vi "LOAD CELL READ.vi"(8 "error in (no error)":errorcluster, 11 "main ref":T1) -> (0 "error out":errorcluster)   [LabVIEW 2025]
uses:
  v06/controls/LAB-IQ UI Data.ctl
  Traction Loop/Traction Receipe Enum.ctl
  v05/LOAD CELL CODE/New Logic/Load cell Enum.ctl
  <vilib>/Analysis/baseanly.llb/Mean (DBL).vi
  <vilib>/Analysis/5stat.llb/RMS (DBL).vi
  <vilib>/Analysis/Matrix/Numeric/Conversions/Array To Matrix - RA.vi
  <vilib>/Analysis/Matrix/Numeric/Conversions/Matrix To Array - RM.vi
  <vilib>/Analysis/NI_AALBase.lvlib
  <vilib>/ptbypt/NI_PtbyPt.lvlib
  <vilib>/Analysis/NI_AALPro.lvlib
  <vilib>/Analysis/Matrix/NI_Matrix.lvlib
panel:
  out "Fload 3":dbl
  out "Fload 2":dbl
  out "Fload":dbl
  out "Friction":dbl
  out "Load Temp":dbl
  out "Zload":dbl
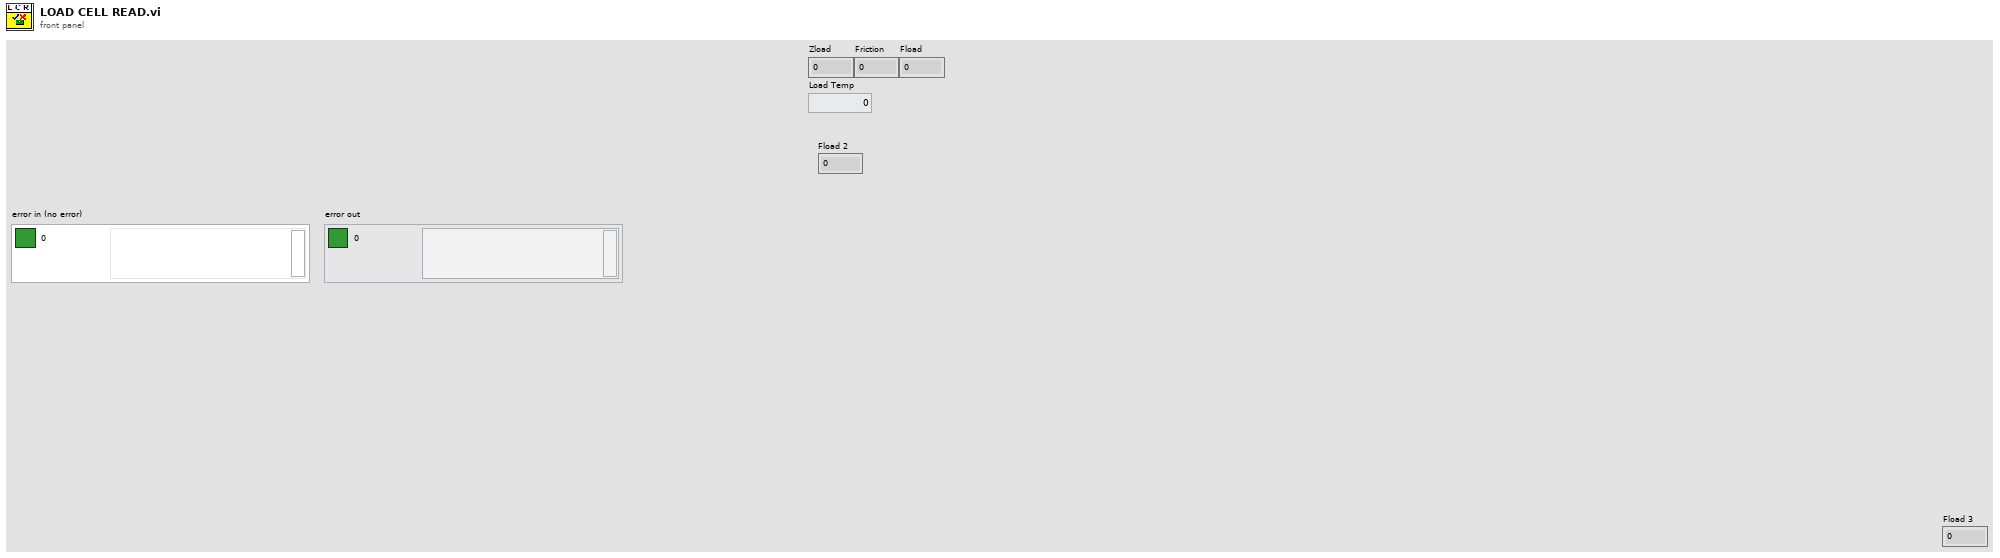
[diagram p1: front panel]
types:
  T1 = typedef "LAB-IQ UI Data.ctl" = cluster{"Main Home Screen":cluster{"GUI":refnum<vi>, "Platform Settings":refnum<vi>, "Configure":refnum<vi>, "Home":refnum<vi>, "EXIT":refnum<vi>, "service 2":refnum<vi>, "MainPage":refnum<vi>, "Analysis":refnum<vi>}, "Platform Settings":cluster{"mm/s  Surge":refnum<vi>, "Drive Error":refnum<vi>, "Disable Axis Jog Soft Limits":refnum<vi>, "mm/s  Sway":refnum<vi>, "Sway and Surge COM Status":refnum<vi>, "Heave COM Status":refnum<vi>, "Enable Platform":refnum<vi>, "Surge Forward Main":refnum<vi>, "Sway Right Main":refnum<vi>, "Sway Left Main":refnum<vi>, "Heave Down Main":refnum<vi>, "Heave Up main":refnum<vi>, "mm/s Heave":refnum<vi>, "mm/sec":refnum<vi>, "mm":refnum<vi>, "Surge Backward Main":refnum<vi>}, "Analysis Screen":cluster{"Analysis Home":refnum<vi>, "Surface Analysis":refnum<vi>, "Imaging":refnum<vi>, "Image Analysis":refnum<vi>, "Post Analysis":refnum<vi>}, "Config Screen":cluster{"Select Load Head":refnum<vi>, "Notes :":refnum<vi>, "FILE":refnum<vi>, "Sample ID :":refnum<vi>, "Operator ID :":refnum<vi>, "Operator Name :":refnum<vi>, "Auto":refnum<vi>}, "Motion Module":cluster{"zNL":refnum<vi>, "NL disp":refnum<vi>, "Rotary Tab":refnum<vi>, "Motion Direction:  3":refnum<vi>, "E.Velocity 2":refnum<vi>, "e.v/ssr 2":refnum<vi>, "Enter Fixed E.Velocity 2":refnum<vi>, "Enter Final SRR 2":refnum<vi>, "Enter initial SRR 2":refnum<vi>, "Enter Fixed SRR 2":refnum<vi>, "Enter the Final E.Velocity (m/s) 2":refnum<vi>, "Enter initial E.Velocity (m/s) 2":refnum<vi>, "Final Speed (RPM) 3":refnum<vi>, "Initial Speed (RPM) 2":refnum<vi>, "Enter the Final Velocity (m/s) 3":refnum<vi>, "Enter initial Velocity (m/s)  3":refnum<vi>, "Ramp Up 2":refnum<vi>, "TEST SELECTION":refnum<vi>, "SPEED SELECTION : ":refnum<vi>, "Angular Oscillation Set":refnum<vi>, "Traction":refnum<vi>, "Step Speed":refnum<vi>, "StepTable For Load-Speed":refnum<vi>, "StepTable For Speed":refnum<vi>, "Surge Forward MM":refnum<vi>, "Surge Backward MM":refnum<vi>, "M3 Image":refnum<vi>, "String 39":refnum<vi>, "Sway Left MM":refnum<vi>, "Sway Right MM":refnum<vi>, "Disable Axis Jog Soft Limits":refnum<vi>, "mm":refnum<vi>, "Heave Down MM":refnum<vi>, "Heave Up MM":refnum<vi>, "Wear Track Diameter (mm)":refnum<vi>, "Set WTD":refnum<vi>, "HomeScratch":refnum<vi>, "HomeRot":refnum<vi>, "PlaceModule":refnum<vi>, "Enter the Angle (Deg)":refnum<vi>, "Enter the Frequency (Hz)":refnum<vi>, "Motion Mode:":refnum<vi>, "LR Sway":refnum<vi>, "Rot Hor":refnum<vi>, "Scratch":refnum<vi>, "LR Cam":refnum<vi>, "MMBack":refnum<vi>, "MMNext":refnum<vi>, "Rot Ver":refnum<vi>, "Rotary Module Selection":refnum<vi>, "calculate rotary":refnum<vi>, "SPEED SELECTION : rotary":refnum<vi>, "Import 2":refnum<vi>, "Save 2":refnum<vi>, "File Path :  2":refnum<vi>, "String 45":refnum<vi>, "StepTable For Speed 3":refnum<vi>, "Enter the Speed(mm/sec)":refnum<vi>, "Enter the Speed(RPM)":refnum<vi>, "Enter Scratch Speed (mm/s):":refnum<vi>, "SwaySpeed Set":refnum<vi>, "Scartch Offset":refnum<vi>, "Motion type:":refnum<vi>, "HomeScratch 2":refnum<vi>, "Enter Scratch length (mm):":refnum<vi>, "Wear Track Diameter":refnum<vi>, "Rotary Speed Exced":refnum<vi>, "Scratch Mode":refnum<vi>, "No of Scratch":refnum<vi>}, "Environmental control":cluster{"Humidity  Status  3":refnum<vi>, "Low Temp  Status  2":refnum<vi>, "TK4 status 2":refnum<vi>, "Stage Temperature":refnum<vi>, "Sample Temperature":refnum<vi>, "Humidity (Amb)":refnum<vi>, "Clear List":refnum<vi>, "Add to list":refnum<vi>, "Wear":refnum<vi>, "Vibration":refnum<vi>, "Humidity (Chamber)":refnum<vi>, "Temperature (Chamber)":refnum<vi>, "ECR ":refnum<vi>, "Temperature (Amb)":refnum<vi>, "Microphone":refnum<vi>, "Acoustic Emission 3":refnum<vi>, "SNext":refnum<vi>, "APBack":refnum<vi>, "Enter the Temperature (°C):":refnum<vi>, "Enter the Stage \nTemperature (°C):":refnum<vi>, "Enter the Humidity (%Rh):":refnum<vi>, "Low Temp":refnum<vi>, "High Temp":refnum<vi>, "Humidity":refnum<vi>, "Sensors Picked":refnum<vi>}, "About Screen":cluster{"Password":refnum<vi>, "Home Service":refnum<vi>, "Advanced Setting":refnum<vi>, "About Tab":refnum<vi>, "ECR Port:":refnum<vi>, "Ramp Port:":refnum<vi>, "Installation/Replacement completed":refnum<vi>, "Loahead":refnum<vi>, "Heave and Surge COM Port:":refnum<vi>, "Sway COM Port:":refnum<vi>, "Temp Modbus:":refnum<vi>, "Humidity Port:":refnum<vi>, "Edit Gain Constants":refnum<vi>, "Save Gain Constants":refnum<vi>}, "Main Screen":cluster{"Main Screen Tab":refnum<vi>, "Angle and Frequency":refnum<vi>, "Stroke (mm)":refnum<vi>, "Angle (Deg)":refnum<vi>, "Main Speed Tab":refnum<vi>, "MTM MOTOR DISPLAY":refnum<vi>, "Disc Speed (m/sec)":refnum<vi>, "Ball Speed (m/sec)":refnum<vi>, "Disc Speed (RPM)":refnum<vi>, "Ball Speed (RPM)":refnum<vi>, "SPEED TAB":refnum<vi>, "Speed (m/sec)":refnum<vi>, "Set Speed (m/sec)":refnum<vi>, "Speed (RPM)":refnum<vi>, "Set Speed":refnum<vi>, "Time Tab":refnum<vi>, "Time ( HH:MM:SS ) 2":refnum<vi>, "Test Duration":refnum<vi>, "Test Duration 4":refnum<vi>, "TEST CYCLE":refnum<vi>, "TOTAL CYCLES":refnum<vi>, "Set Load (N)":refnum<vi>, "Temp Tabs":refnum<vi>, "Heater":refnum<vi>, "TK4 status":refnum<vi>, "ChamberTemp":refnum<vi>, "SetTmp":refnum<vi>, "Controller  Status":refnum<vi>, "ChamberTemp 2":refnum<vi>, "SetTmp 2":refnum<vi>, "Controller  Status 2":refnum<vi>, "ChamberTemp 3":refnum<vi>, "SetTmp 3":refnum<vi>, "Cooling":refnum<vi>, "Load Communication":refnum<vi>, "Ambient \nTemperature":refnum<vi>, "HumCOMStatus":refnum<vi>, "Ambient\n Humidity":refnum<vi>, "Freq (Hz)":refnum<vi>, "Load En":refnum<vi>, "NLt":refnum<vi>, "zNL 2":refnum<vi>, "Humidity On":refnum<vi>, "humidity disp":refnum<vi>, "Set Humidity":refnum<vi>, "NL disp 2":refnum<vi>, "Humidity On 2":refnum<vi>, "humidity disp 2":refnum<vi>, "Set Humidity 2":refnum<vi>, "NL disp 3":refnum<vi>, "AppLoadSeq scratch":refnum<vi>, "Stop Scratch":refnum<vi>, "ClrLog":refnum<vi>, "Trip Log":refnum<vi>, "STOP":refnum<vi>, "Start Test":refnum<vi>, "Test status":refnum<vi>, "AR Led":refnum<vi>, "Data":refnum<vi>, "Health":refnum<vi>, "Sway COM Status":refnum<vi>, "Heave COM Status":refnum<vi>, "Grp Tab":refnum<vi>, "Sub Graph":refnum<vi>, "SD (mm)":refnum<vi>, "Siliding distance Reset Graph":refnum<vi>, "SDGp":refnum<vi>, "Humidity Reset Graph":refnum<vi>, "HumrGp":refnum<vi>, "Acoustic Emission (mV)":refnum<vi>, "Aqucostic Reset Graph":refnum<vi>, "gACQUOS":refnum<vi>, "ECR RESET":refnum<vi>, "ECR":refnum<vi>, "Temperature Reset":refnum<vi>, "Acoustic Emission (mV) 2":refnum<vi>, "Aqucostic Reset Graph 2":refnum<vi>, "gACQUOS 2":refnum<vi>, "ECR RESET 2":refnum<vi>, "ECR 2":refnum<vi>, "Temperature Reset 2":refnum<vi>, "Temperature (deg c)":refnum<vi>, "Speed Reset Graph":refnum<vi>, "Speed Tab":refnum<vi>, "MTM DISC  SPEED":refnum<vi>, "MTM BALL SPEED":refnum<vi>, "speed mm/sec":refnum<vi>, "Hymidity":refnum<vi>, "Humidity Disable trip":refnum<vi>, "CoF Trip  2":refnum<vi>, "Depth Trip":refnum<vi>, "Weart Deapth":refnum<vi>, "Depth Reset Graph":refnum<vi>, "Weart":refnum<vi>, "Depthz":refnum<vi>, "Depth (µm)":refnum<vi>, "WearGp":refnum<vi>, "NL Trip 2":refnum<vi>, "Load pid":refnum<vi>, "Load Disable Trip":refnum<vi>, "Load Reset Graph":refnum<vi>, "NL Display 4":refnum<vi>, "Main Chart 3":refnum<vi>, "BACK":refnum<vi>, "Depth Trip 2":refnum<vi>, "COF TRIP ":refnum<vi>, "Friction Force (N)":refnum<vi>, "FF Reset Graph":refnum<vi>, "FF Disable Trip":refnum<vi>, "FF TRIP":refnum<vi>, "COF Disable Trip":refnum<vi>, "COF Reset Graph":refnum<vi>, "Start Test Temp":refnum<vi>, "zFF":refnum<vi>, "Friction Force (N) Graph":refnum<vi>, "Coefficient of Friction":refnum<vi>, "Scratch Start Test":refnum<vi>, "FF Tab":refnum<vi>, "Cyclic Friction Force (N)":refnum<vi>, "CZ FF":refnum<vi>, "Cyclic Friction Force (N) Graph":refnum<vi>, "Cyclic Coefficient of Friction":refnum<vi>, "Cyclic FF TRIP":refnum<vi>, "Cyclic FF Disable Trip":refnum<vi>, "cyclic COF Disable Trip":refnum<vi>, "cyclic COF TRIP":refnum<vi>, "cyclic COF Reset Graph":refnum<vi>, "Cyclic FF Reset Graph":refnum<vi>, "Test Trip":refnum<vi>, "Multi Scratch Pass":refnum<vi>, "Scratch Start Recording":refnum<vi>, "Coefficient of Friction 2":refnum<vi>, "Acoustic Emission":refnum<vi>, "Friction Force (N) 2":refnum<vi>, "Depth (Microns)":refnum<vi>, "Normal Load ( N )":refnum<vi>}, "Loading":cluster{"Indentation":refnum<vi>, "Reference Sample":refnum<vi>, "Load Cell Communication Slide":refnum<vi>, "com 3":refnum<vi>, "com":refnum<vi>, "DecaForce COM Status":refnum<vi>, "Update":refnum<vi>, "Clear 3":refnum<vi>, "seq":refnum<vi>, "Stribeck table":refnum<vi>, "Stribeck Table  For loading":refnum<vi>, "Loading Mode":refnum<vi>, "Enter the Final Load (N)":refnum<vi>, "Enter the CoF Trip":refnum<vi>, "Enter the Friction Force Trip":refnum<vi>, "Enter the Normal load Trip":refnum<vi>, "Enter the Load  (N)":refnum<vi>, "KiloForce":refnum<vi>, "DecaForce ":refnum<vi>, "MicroForce":refnum<vi>, "LHBack":refnum<vi>, "LHNext":refnum<vi>, "Enter the Loading Rate (N/min)":refnum<vi>, "Message":refnum<vi>, "Warning 2":refnum<vi>, "SSP 0.75":refnum<vi>, "SSP 0.5":refnum<vi>, "SSP 0.3":refnum<vi>, "Warning":refnum<vi>, "gui GIF":refnum<vi>, "Communication is established":refnum<vi>, "AppLoad 4":refnum<vi>, "Multipoint":refnum<vi>, "Load Selection":refnum<vi>}, "PID":cluster{"Ramp":refnum<vi>, "Vertical load (N)":refnum<vi>, "apply load":refnum<vi>, "apply load 2":refnum<vi>, "Enter ByPass Load":refnum<vi>, "Bypass Load":refnum<vi>, "gFF Rot":refnum<vi>}, "Config Parameters":cluster{"Tab Control 3":refnum<vi>, "Tab Control 19":refnum<vi>, "SAMPLES":refnum<vi>, "Re-initilaize":refnum<vi>, "Filter ON/OFF":refnum<vi>, "TracHomeSurgeOffsetCounts 10MM":refnum<vi>, "TracHomeSwayOffsetCounts 10MM":refnum<vi>, "Acoustic Emission:":refnum<vi>, "Apply Filter (FF)":refnum<vi>, "Filter% 2":refnum<vi>, "Apply Filter (Load)":refnum<vi>, "Filter% ":refnum<vi>, "Sway distance (mm)":refnum<vi>, "Surge distance (mm)":refnum<vi>, "DataSavingLoopDelay(ms)":refnum<vi>, "SAVE 2":refnum<vi>, "Enter Distance":refnum<vi>, "Sway Counts:":refnum<vi>, "Distance (mm): 3":refnum<vi>, "Surge Counts:":refnum<vi>, "Distance (mm): 2":refnum<vi>, "Distance (mm):":refnum<vi>, "Heave Counts:":refnum<vi>, "LRMHomeSurgeOffsetCounts":refnum<vi>, "LRMHomeSwayOffsetCounts":refnum<vi>, "TracHomeSurgeOffsetCounts 20MM":refnum<vi>, "TracHomeSwayOffsetCounts 20MM":refnum<vi>, "RotHomeSwayOffsetCounts":refnum<vi>, "RotHomeSurgeOffsetCounts":refnum<vi>, "Heave distance":refnum<vi>, "Zmm":refnum<vi>, "Heave Pulses/mm":refnum<vi>, "Surge Pulses/mm":refnum<vi>, "Sway Pulses/mm":refnum<vi>, "Heave Pitch":refnum<vi>, "Surge Pitch":refnum<vi>, "Sway Pitch":refnum<vi>, "Heave PPR":refnum<vi>, "Surge PPR":refnum<vi>, "Sway PPR":refnum<vi>, "Tab Control 5":refnum<vi>, "Tab Control 14":refnum<vi>, "Tab Control 26":refnum<vi>, "AE":refnum<vi>, "Heave Loop Delay":refnum<vi>, "Heave PID Speed":refnum<vi>, "Surge Jog Speed":refnum<vi>, "Heave Jog Speed":refnum<vi>, "Sway Loop Delay":refnum<vi>, "Sway PID Speed":refnum<vi>, "Sway Jog Speed":refnum<vi>, "DEPTH TRIP VALUE":refnum<vi>, "LOAD TRIP VALUE":refnum<vi>, "DEPTH TRIP   ENABLE":refnum<vi>, "LOAD TRIP  ENABLE":refnum<vi>, "CYCLIC FF TRIP VALUE":refnum<vi>, "FF TRIP VALUE":refnum<vi>, "CYCLIC CoF TRIP VALUE":refnum<vi>, "COF TRIP VALUE":refnum<vi>, "CYCLIC COF TRIP  ENABLE":refnum<vi>, "CYCLIC FF TRIP  ENABLE":refnum<vi>, "FF TRIP  ENABLE":refnum<vi>, "COF TRIP  ENABLE":refnum<vi>, "JOG TRIP LOAD VALUE (N)":refnum<vi>, "Rotary Vertical":refnum<vi>, "Traction":refnum<vi>, "Scratch":refnum<vi>, "LRM CAM":refnum<vi>, "Sway LRM":refnum<vi>, "Rotary Horizontal":refnum<vi>, "SURGE SPEED":refnum<vi>, "SURGE BACKWARD COUNT":refnum<vi>, "SURGE FORWARD COUNT":refnum<vi>, "Start Button":refnum<vi>}, "Loading Com Port":cluster{"ClearAll":refnum<vi>, "Mz(Nm)":refnum<vi>, "My(Nm)":refnum<vi>, "Mx(Nm)":refnum<vi>, "Save Dwell":refnum<vi>, "Acq Delay (ms)":refnum<vi>, "Burst Delay (ms)":refnum<vi>, "model":refnum<vi>, "SN":refnum<vi>, "FFx(N)":refnum<vi>, "Sensor IP":refnum<vi>, "Port":refnum<vi>, "FFy(N)":refnum<vi>, "Load(N)":refnum<vi>, "delete Handle":refnum<vi>, "Create Handle":refnum<vi>, "ft_data":refnum<vi>, "ft_range":refnum<vi>, "ft_data 2":refnum<vi>, "stop 6":refnum<vi>, "running_flag":refnum<vi>, "ft_udp_handle":refnum<vi>, "get-data-return":refnum<vi>, "get-range-return":refnum<vi>, "zero-return":refnum<vi>, "filter-return":refnum<vi>, "initial-return":refnum<vi>, "deleteHandle-result":refnum<vi>, "Load Cell Temp":refnum<vi>, "Load Cell":refnum<vi>, "ZeroAll":refnum<vi>, "FORCE (N)":refnum<vi>, "TORQUE (N-m)":refnum<vi>, "Load Cell Link":refnum<vi>}, "Heave AND Surge":cluster{"SURGE POSE":refnum<vi>, "error out Read":refnum<vi>, "HEAVE POSE":refnum<vi>, "State":refnum<vi>, "Homed":refnum<vi>, "Sequence ID":refnum<vi>, "error out Write":refnum<vi>, "faultCode":refnum<vi>, "Ack ID":refnum<vi>, "SPEED":refnum<vi>, "Distance":refnum<vi>, "Mode Command":refnum<vi>, "Heave and Surge Read":refnum<vi>, "Read Heave Temp":refnum<vi>, "Spare 15":refnum<vi>, "Spare 14":refnum<vi>, "Spare 13":refnum<vi>, "Spare 12":refnum<vi>, "Spare 11":refnum<vi>, "Spare 10":refnum<vi>, "Spare 9":refnum<vi>, "Spare 8":refnum<vi>, "Spare 7":refnum<vi>, "Spare 4":refnum<vi>, "Spare 3":refnum<vi>, "Spare 2":refnum<vi>, "Humidity":refnum<vi>, "Temp":refnum<vi>, "Node Id":refnum<vi>, "Spare 1":refnum<vi>, "SPARE 4":refnum<vi>, "SPARE 3":refnum<vi>, "SPARE 2":refnum<vi>, "SPARE 1":refnum<vi>, "fwMajor":refnum<vi>, "fwMinor":refnum<vi>, "Manual Write":refnum<vi>, "Heave and Surge Write":refnum<vi>, "SPARE 5":refnum<vi>, "Reserved ":refnum<vi>, "SPARE 8":refnum<vi>, "SPARE 6":refnum<vi>, "SPARE 7":refnum<vi>, "SPARE 17":refnum<vi>, "SPARE 16":refnum<vi>, "SPARE 15":refnum<vi>, "SPARE 14":refnum<vi>, "SPARE 13":refnum<vi>, "SPARE 12":refnum<vi>, "SPARE 11":refnum<vi>, "SPARE 10":refnum<vi>, "SPARE 9":refnum<vi>, "System UPTIME":refnum<vi>, "Missed Packets":refnum<vi>, "faultCode Surge Right":refnum<vi>, "faultCode Surge Left":refnum<vi>, "faultCode Heave":refnum<vi>, "UPLINK HEAVE":refnum<vi>, "DOWNLINK HEAVE":refnum<vi>}, "New PID LOGIC":cluster{"Fine Tune Zone":refnum<vi>, "PID SDelay":refnum<vi>, "Max_pos_limit":refnum<vi>, "Min_pos_limit":refnum<vi>, "i_limit":refnum<vi>, "pct_scale":refnum<vi>, "Deadband":refnum<vi>, "Kd":refnum<vi>, "Ki":refnum<vi>, "Kp":refnum<vi>, "Current Position":refnum<vi>, "Set Load":refnum<vi>, "Current Load":refnum<vi>, "Pulse delta":refnum<vi>, "Init Step":refnum<vi>, "Max Step Linit":refnum<vi>, "min_deadband_floor":refnum<vi>, "dynamic_spindle_noise_scalar":refnum<vi>, "min_finetune_floor":refnum<vi>, "filter_alpha":refnum<vi>, "PID":refnum<vi>}, "SWAY ":cluster{"fwMajor":refnum<vi>, "Homed":refnum<vi>, "Rotary POSE":refnum<vi>, "State":refnum<vi>, "SWAY POSE":refnum<vi>, "Ack ID":refnum<vi>, "faultCode":refnum<vi>, "Node Id":refnum<vi>, "fwMinor":refnum<vi>, "Spare 6":refnum<vi>, "Spare 5":refnum<vi>, "Spare 4":refnum<vi>, "Spare 3":refnum<vi>, "Spare 2":refnum<vi>, "Spare 1":refnum<vi>, "Spare 7":refnum<vi>, "SPARE  5":refnum<vi>, "error out Write  SWAY ":refnum<vi>, "error out Read SWAY ":refnum<vi>, "Manual Write SWAY ":refnum<vi>, "SWAY WRITE":refnum<vi>, "SPARE  4":refnum<vi>, "SPARE  3":refnum<vi>, "SPARE 2":refnum<vi>, "SPARE 1":refnum<vi>, "Spare 15":refnum<vi>, "Spare 14":refnum<vi>, "Spare 13":refnum<vi>, "Spare 12":refnum<vi>, "Spare 11":refnum<vi>, "Spare 9":refnum<vi>, "Spare 8":refnum<vi>, "SPEED":refnum<vi>, "Distance":refnum<vi>, "Mode Command":refnum<vi>, "Sequence ID":refnum<vi>, "SWAY READ":refnum<vi>, "Spare 10":refnum<vi>, "Read SWAY Temp":refnum<vi>, "faultCode Sway ":refnum<vi>, "Missed Packets":refnum<vi>, "System UPTIME sway":refnum<vi>, "SPARE 6":refnum<vi>, "SPARE 7":refnum<vi>, "SPARE 9":refnum<vi>, "SPARE 11":refnum<vi>, "SPARE 10":refnum<vi>, "SPARE 8":refnum<vi>, "SPARE 13":refnum<vi>, "SPARE 12":refnum<vi>, "SPARE 17":refnum<vi>, "SPARE 16":refnum<vi>, "SPARE 15":refnum<vi>, "SPARE 14":refnum<vi>, "Reserved":refnum<vi>, "faultCode Rotary":refnum<vi>, "UPLINK SWAY":refnum<vi>, "DOWNLINK SWAY":refnum<vi>}, "Analysis Screen":cluster{"Analysis Home":refnum<vi>, "Refresh 2":refnum<vi>, "MEAN 4":refnum<vi>, "SD 4":refnum<vi>, "VARIANCE 4":refnum<vi>, "MEAN  3":refnum<vi>, "SD  3":refnum<vi>, "VARIANCE  3":refnum<vi>, "MEAN 2":refnum<vi>, "SD  2":refnum<vi>, "VARIANCE 2":refnum<vi>, "MEAN":refnum<vi>, "SD":refnum<vi>, "VARIANCE":refnum<vi>, "File 4 Discription":refnum<vi>, "OPEN 4":refnum<vi>, "File Name 4":refnum<vi>, "OPEN 3":refnum<vi>, "File 3 Discription":refnum<vi>, "File Name 3":refnum<vi>, "Y-AXIS":refnum<vi>, "X-AXIS":refnum<vi>, "XY Graph":refnum<vi>, "File Name 2":refnum<vi>, "File Name 1":refnum<vi>, "OPEN 2":refnum<vi>, "OPEN 1":refnum<vi>, "File 1 Discription ":refnum<vi>, "File 2 Discription":refnum<vi>, "Export":refnum<vi>, "File Format":refnum<vi>}, "Traction":cluster{"faultCode Traction 2":refnum<vi>, "faultCode Traction 1":refnum<vi>, "Missed Packets":refnum<vi>, "System UPTIME Traction":refnum<vi>, "SPARE 17":refnum<vi>, "SPARE 16":refnum<vi>, "SPARE 15":refnum<vi>, "SPARE 14":refnum<vi>, "SPARE 13":refnum<vi>, "SPARE 12":refnum<vi>, "SPARE 11":refnum<vi>, "SPARE 10":refnum<vi>, "SPARE 9":refnum<vi>, "SPARE 8":refnum<vi>, "SPARE 7":refnum<vi>, "SPARE 6":refnum<vi>, "Reserved":refnum<vi>, "SPARE  5":refnum<vi>, "Manual Write TRACTION":refnum<vi>, "TRACTION WRITE":refnum<vi>, "SPARE  4":refnum<vi>, "SPARE  3":refnum<vi>, "SPARE 2":refnum<vi>, "SPARE 1":refnum<vi>, "Spare 7":refnum<vi>, "Spare 6":refnum<vi>, "Spare 5":refnum<vi>, "Spare 4":refnum<vi>, "Spare 2":refnum<vi>, "Spare 1":refnum<vi>, "Node Id":refnum<vi>, "Read TRACTION Temp":refnum<vi>, "fwMinor":refnum<vi>, "fwMajor":refnum<vi>, "faultCode":refnum<vi>, "TRACTION POSE":refnum<vi>, "TRACTION POSE 2":refnum<vi>, "Homed":refnum<vi>, "State":refnum<vi>, "Ack ID":refnum<vi>, "SPEED":refnum<vi>, "Distance":refnum<vi>, "Mode Command":refnum<vi>, "Sequence ID":refnum<vi>, "error out Read TRACTION":refnum<vi>, "error out Write  TRACTION":refnum<vi>, "TRACTION READ":refnum<vi>, "Spare 3":refnum<vi>, "Downlink traction":refnum<vi>, "Uplink Traction":refnum<vi>}, "Traction reciepe":cluster{"SRR Sweep Range (%) Stribeck":refnum<vi>, "Traction Receipe":refnum<vi>, "Total Execution Time":refnum<vi>, "Total Steps":refnum<vi>, "Duration / Step (s)  Stribeck":refnum<vi>, "STRIBECK Fixed SRR List (%)":refnum<vi>, "Duration / Step (s) Traction":refnum<vi>, "SRR Sweep Range (%) traction":refnum<vi>, "Rolling Speed (mm/s)":refnum<vi>, "Temperature Stages (°C)":refnum<vi>, "Ball Load (N)":refnum<vi>, "Lubricant Name":refnum<vi>, "Profile File Name":refnum<vi>, "SET entrainment Velocity":refnum<vi>, "Test Array Size":refnum<vi>, "SRR INDEX [ STRIBECK]":refnum<vi>, "Stribeck Size":refnum<vi>, "SET SRR":refnum<vi>, "ELAPSED TIMER ":refnum<vi>, "BALL SET RPM":refnum<vi>, "DISC SET RPM":refnum<vi>, "SET LOAD":refnum<vi>, "TEMPERATURE READ":refnum<vi>, "SET TEMPERATURE":refnum<vi>, "Traction Size":refnum<vi>, "DISC SPEED (rpm)":refnum<vi>, "BALL SPEED (rpm)":refnum<vi>, "BALL WEAR TRACK":refnum<vi>, "DISC WEARTRACK":refnum<vi>, "SRR INDEX [ TRACTION]":refnum<vi>, "Start Index Type":refnum<vi>, "Enum - Menu":refnum<vi>, "Ball (mm/sec)":refnum<vi>, "Disc (mm/sec)":refnum<vi>, "Traction Receipe Update Details":refnum<vi>}, "Traction Control":cluster{"HomeTraction":refnum<vi>, "Demo Mode Display":refnum<vi>, "Traction Message":refnum<vi>, "Traction Step Update Details":refnum<vi>, "Main Tab sequence for selection":refnum<vi>, "Ramp Tab":refnum<vi>, "e.v/ssr":refnum<vi>, "Enter Fixed E.Velocity":refnum<vi>, "Enter Final SRR":refnum<vi>, "Enter initial SRR":refnum<vi>, "Enter Fixed SRR":refnum<vi>, "Enter the Final E.Velocity (m/s)":refnum<vi>, "Enter initial E.Velocity (m/s)":refnum<vi>, "Ball WTD":refnum<vi>, "E.Velocity":refnum<vi>, "Enter the Final Velocity (m/s)":refnum<vi>, "Enter initial Velocity (m/s)":refnum<vi>, "Ramp Up   Disc":refnum<vi>, "Initial DiscSpeed (RPM)":refnum<vi>, "Final Speed (RPM) Ball":refnum<vi>, "Final Speed (RPM)":refnum<vi>, "Initial Speed (RPM) Ball":refnum<vi>, "Enter the Final Velocity (m/s) Ball":refnum<vi>, "Enter initial Velocity (m/s) Ball":refnum<vi>, "Ramp Up":refnum<vi>, "ExceedBallSpeed step":refnum<vi>, "ExceedDiscSpeed":refnum<vi>, "BallSpeed Exceed Indication":refnum<vi>, "Apply":refnum<vi>, "SPEED SELECTION : MTM":refnum<vi>, "SPEED SELECTION : MTM 2":refnum<vi>, "TEST SELECTION (MTM)":refnum<vi>, "MTM Test Selection":refnum<vi>, "File Path Tab":refnum<vi>, "File Path String":refnum<vi>, "Save":refnum<vi>, "Save  2":refnum<vi>, "Import ":refnum<vi>, "File Path :":refnum<vi>, "Step Sequence Indication Tab":refnum<vi>, "Step Sequence Indication":refnum<vi>, "Calculate Step":refnum<vi>, "StepTable":refnum<vi>, "ExceedDiscSpeed  Cinstant Speed":refnum<vi>, "ExceedBallSpeed Constant":refnum<vi>, "TEST SELECTION (MTM) 2":refnum<vi>, "SPEED SELECTION : MTM 3":refnum<vi>, "MTM Test Selection 2":refnum<vi>, "Enter the Speed (m/sec): ":refnum<vi>, "Enter the Speed (m/sec):  2":refnum<vi>, "Enter the Speed (RPM):":refnum<vi>, "Lower Spped ":refnum<vi>, "Upper":refnum<vi>, "Enter the Speed (RPM):Ball":refnum<vi>, "Disc Motion Direction: ":refnum<vi>, "Ball Motion Direction :":refnum<vi>, "Motion Mode: ":refnum<vi>, "Wear Track Diameter (mm) ":refnum<vi>, "Disc Speed Indicator":refnum<vi>, "ExceedBallSpeed":refnum<vi>}, "Acquostic":cluster{"Last Config Rejected ":refnum<vi>, "rx command count":refnum<vi>, "Current Filter Id":refnum<vi>, "Isolated Gain":refnum<vi>, "DAQ Status":refnum<vi>, "error out":refnum<vi>, "error in (no error)":refnum<vi>, "Uplink Packet":refnum<vi>, "data out":refnum<vi>, "Downlink Packet":refnum<vi>, "Gains":refnum<vi>, "Manual Write Acquostic":refnum<vi>, "Acoustic Graphs":refnum<vi>}, "ABOUT":cluster{"version":refnum<vi>, "Operating System":refnum<vi>, "Version":refnum<vi>, "Workorder":refnum<vi>, "Runtime":refnum<vi>, "Instrument Serial":refnum<vi>, "Firmware Version":refnum<vi>, "Info":refnum<vi>}, "Temperature Port":cluster{"Temperature":refnum<vi>, "error out Temperature":refnum<vi>, "READ TEMPERATURE":refnum<vi>}}
  T2 = cluster{"model":string, "SN":i32, "Sensor IP":string, "Port":i32, "Acq Delay (ms)":dbl, "Burst Delay (ms)":dbl, "Save Dwell":dbl, "FORCE (N)":dbl[][], "TORQUE (N-m)":dbl[][], "ft_data":dbl[], "running_flag":bool, "ClearAll":bool, "ZeroAll":bool}
  T3 = typedef "Load cell Enum.ctl" = enum16{"Init", "set UDP", "Read Info", "set Low Pass Filter", "Set Zero", "get data", "close", "REInit"}
  T4 = typedef "NI_Matrix.lvlib/RealMatrix.ctl" = dbl[][]
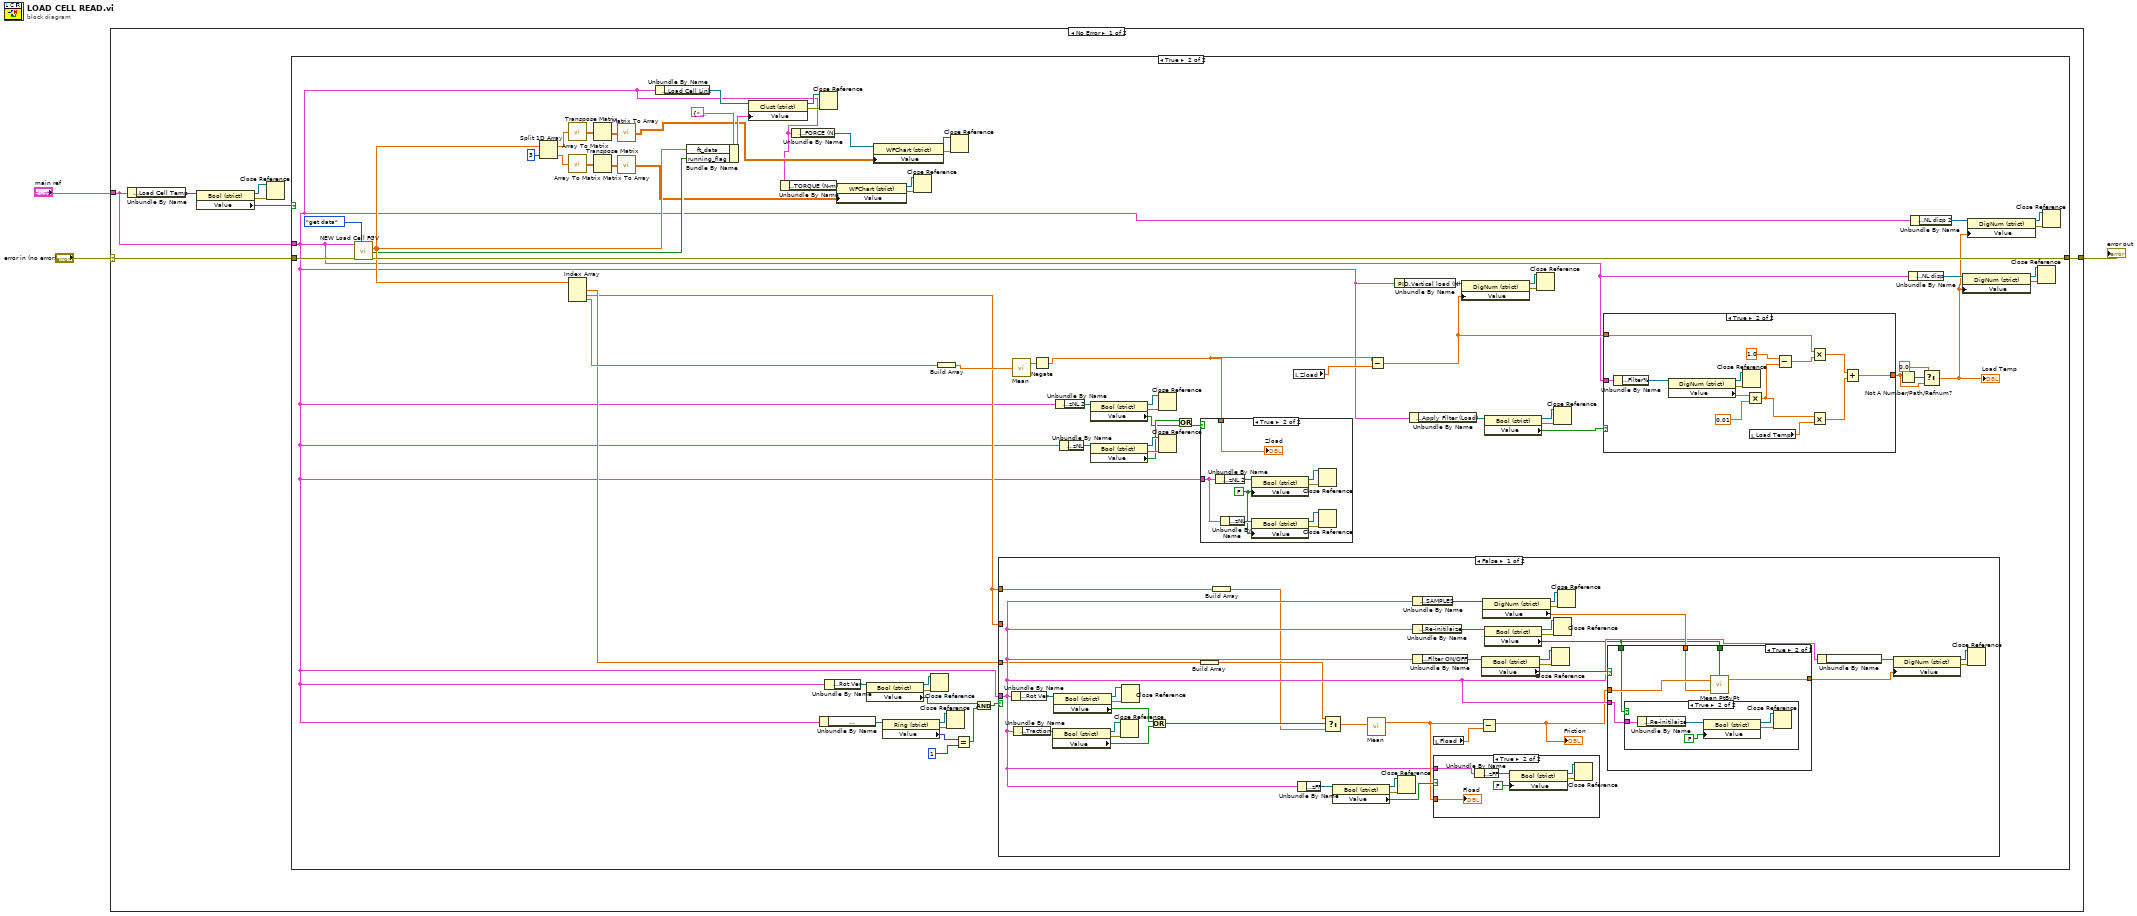
[diagram p0: block diagram]
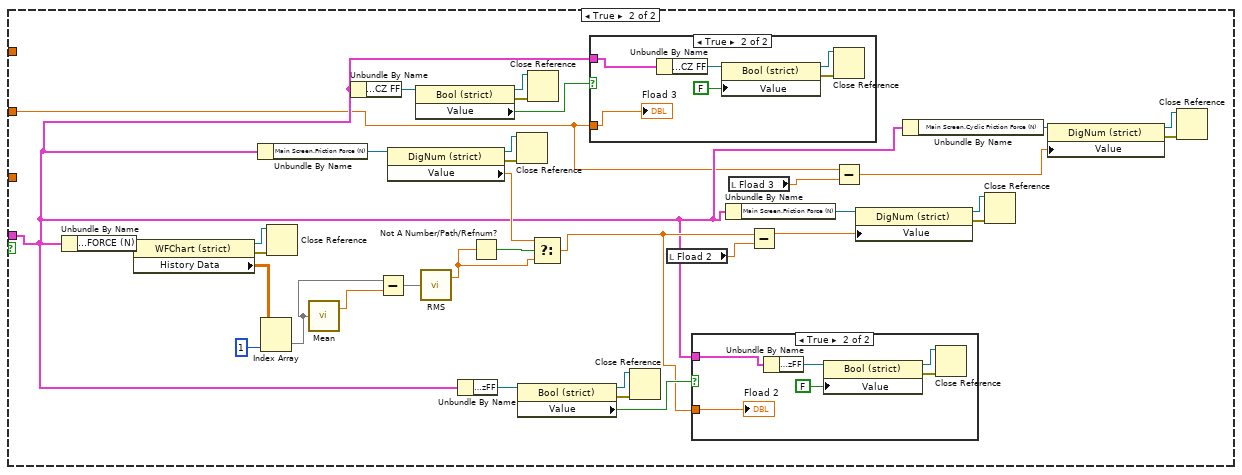
[diagram p6: hidden frame]
diagram:
  n1 = case shown="No Error" "error in (no error)" {
    selector: "error in (no error)" -> [w6 _]
    tunnel: "main ref" -> [w4 _]
    tunnel: [w5 _] -> w1
    frame No Error {
      n2 = Unbundle By Name(w4) -> ("Loading Com Port.Load Cell Temp"=w8:refnum<vi>)
      n3 = property class="Bool (strict)"(reference=w8) -> (reference out=w10:refnum<vi>, error out=w9:errorcluster, "Value"=w7:bool)  [unwired: 1 in]
      n4 = Close Reference(reference=w10, error in (no error)=w9) -> ()  [unwired: 1 out]
      n5 = case shown="True" w7 {
        tunnel: w6 -> [w11 w82]
        tunnel: [w11 w81] -> w5
        tunnel: w4 -> [_ w13]
        frame False {
        }
        frame True {
          n6 = call "NEW Load Cell FGV.vi"("Enum - Menu"=Load_cell_Enum."get data", "error in (no error)"=w82, "main ref"=w13) -> ("error out"=w81:errorcluster, "Running Flag"=w21:bool, "FT Data"=w22:dbl[])  [unwired: 6 in]
          n7 = Split 1D Array(array=w22, index=3) -> (first subarray=w36:dbl[], second subarray=w33:dbl[])
          n8 = call-poly <vilib>:"Array To Matrix.vi"("Real 1D Array"=w36) -> ("Real Matrix (Column Vector)"=w38:T4)
          n9 = call-poly <vilib>:"Array To Matrix.vi"("Real 1D Array"=w33) -> ("Real Matrix (Column Vector)"=w35:T4)
          n10 = Index Array(array=w22) -> (element #1=w29:dbl, element #2=w28:dbl, element #3=w32:dbl)  [unwired: 3 in]
          n11 = Transpose Matrix(1:w38) -> (0:w37:T4)
          n12 = Transpose Matrix(1:w35) -> (0:w34:T4)
          n13 = call-poly <vilib>:"Matrix To Array.vi"("Real Matrix"=w37) -> ("Real 2D Array"=w19:dbl[][])
          n14 = call-poly <vilib>:"Matrix To Array.vi"("Real Matrix"=w34) -> ("Real 2D Array"=w12:dbl[][])
          n15 = Unbundle By Name(w13) -> ("Loading Com Port.Load Cell Link"=w27:refnum<vi>)
          n16 = Bundle By Name(cluster=T2 {"model"="", "SN"=0, "Sensor IP"="", "Port"=0, "Acq Delay (ms)"=0.0, "Burst Delay (ms)"=0.0, "Save Dwell"=0.0, "FORCE (N)"=[], "TORQUE (N-m)"=[], "ft_data"=[], "running_flag"=FALSE, "ClearAll"=FALSE, "ZeroAll"=FALSE} ("Value"), "ft_data"=w22, "running_flag"=w21) -> (w23:T2)
          n17 = property class="Clust (strict)"(reference=w27, "Value"=w23) -> (reference out=w25:refnum<vi>, error out=w26:errorcluster)  [unwired: 1 in]
          n18 = Unbundle By Name(w13) -> ("Loading Com Port.TORQUE (N-m)"=w16:refnum<vi>)
          n19 = Unbundle By Name(w13) -> ("Loading Com Port.FORCE (N)"=w20:refnum<vi>)
          n20 = Close Reference(reference=w25, error in (no error)=w26) -> ()  [unwired: 1 out]
          n21 = Unbundle By Name(w13) -> ("Motion Module.Motion Mode:"=w45:refnum<vi>)
          n22 = Unbundle By Name(w13) -> ("Motion Module.Rot Ver"=w50:refnum<vi>)
          n23 = property class="WFChart (strict)"(reference=w16, "Value"=w12) -> (reference out=w15:refnum<vi>, error out=w14:errorcluster)  [unwired: 1 in]
          n24 = property class="Bool (strict)"(reference=w50) -> (reference out=w48:refnum<vi>, error out=w49:errorcluster, "Value"=w42:bool)  [unwired: 1 in]
          n25 = property class="WFChart (strict)"(reference=w20, "Value"=w19) -> (reference out=w18:refnum<vi>, error out=w17:errorcluster)  [unwired: 1 in]
          n26 = property class="Ring (strict)"(reference=w45) -> (reference out=w47:refnum<vi>, error out=w46:errorcluster, "Value"=w44:u16)  [unwired: 1 in]
          n27 = Close Reference(reference=w15, error in (no error)=w14) -> ()  [unwired: 1 out]
          n28 = Close Reference(reference=w48, error in (no error)=w49) -> ()  [unwired: 1 out]
          n29 = Build Array(w32) -> (w31:dbl[])
          n30 = Close Reference(reference=w47, error in (no error)=w46) -> ()  [unwired: 1 out]
          n31 = Close Reference(reference=w18, error in (no error)=w17) -> ()  [unwired: 1 out]
          n32 = Equal?(x=w44, y=u16 1) -> (x = y?=w41:bool)
          n33 = And(x=w42, y=w41) -> (x .and. y?=w40:bool)
          n34 = case shown="False" w40 {
            tunnel: w13 -> [w91 w145]
            tunnel: w28 -> [_ w139]
            tunnel: w29 -> [w86 _]
            tunnel: w28 -> [w85 _]
            frame False {
              n35 = Unbundle By Name(w91) -> ("Motion Module.Rot Ver"=w113:refnum<vi>)
              n36 = Unbundle By Name(w91) -> ("Motion Module.Traction"=w118:refnum<vi>)
              n37 = property class="Bool (strict)"(reference=w118) -> (reference out=w116:refnum<vi>, error out=w117:errorcluster, "Value"=w120:bool)  [unwired: 1 in]
              n38 = property class="Bool (strict)"(reference=w113) -> (reference out=w115:refnum<vi>, error out=w114:errorcluster, "Value"=w119:bool)  [unwired: 1 in]
              n39 = Close Reference(reference=w116, error in (no error)=w117) -> ()  [unwired: 1 out]
              n40 = Close Reference(reference=w115, error in (no error)=w114) -> ()  [unwired: 1 out]
              n41 = Or(x=w119, y=w120) -> (x .or. y?=w112:bool)
              n42 = Build Array(w86) -> (w84:dbl[])
              n43 = Build Array(w85) -> (w83:dbl[])
              n44 = Unbundle By Name(w91) -> ("Main Screen.zFF"=w110:refnum<vi>)
              n45 = Select(t=w84, s=w112, f=w83) -> (s? t:f=w111:dbl[])
              n46 = property class="Bool (strict)"(reference=w110) -> (reference out=w108:refnum<vi>, error out=w109:errorcluster, "Value"=w107:bool)  [unwired: 1 in]
              n47 = call-poly <vilib>:"Mean.vi"("X"=w111) -> ("mean"=w99:dbl)  [unwired: 1 out]
              n48 = Close Reference(reference=w108, error in (no error)=w109) -> ()  [unwired: 1 out]
              n49 = Unbundle By Name(w91) -> ("Config Parameters.SAMPLES"=w98:refnum<vi>)
              n50 = Unbundle By Name(w91) -> ("Config Parameters.Re-initilaize"=w100:refnum<vi>)
              n51 = Unbundle By Name(w91) -> ("Config Parameters.Filter ON/OFF"=w106:refnum<vi>)
              n52 = case shown="True" w107 {
                tunnel: w91 -> [_ w135]
                tunnel: w99 -> [_ w133]
                frame False {
                }
                frame True {
                  n53 = Unbundle By Name(w135) -> ("Main Screen.zFF"=w136:refnum<vi>)
                  n54 = property class="Bool (strict)"(reference=w136, "Value"=FALSE) -> (reference out=w138:refnum<vi>, error out=w137:errorcluster)  [unwired: 1 in]
                  n55 = Close Reference(reference=w138, error in (no error)=w137) -> ()  [unwired: 1 out]
                  "Fload" <- w133
                }
              }
              n56 = local read "Fload"() -> (w87:dbl)
              n57 = Subtract(x=w99, y=w87) -> (x-y=w88:dbl)
              "Friction" <- w88
              n58 = property class="Bool (strict)"(reference=w106) -> (reference out=w104:refnum<vi>, error out=w105:errorcluster, "Value"=w103:bool)  [unwired: 1 in]
              n59 = property class="DigNum (strict)"(reference=w98) -> (reference out=w96:refnum<vi>, error out=w97:errorcluster, "Value"=w95:dbl)  [unwired: 1 in]
              n60 = property class="Bool (strict)"(reference=w100) -> (reference out=w102:refnum<vi>, error out=w101:errorcluster, "Value"=w89:bool)  [unwired: 1 in]
              n61 = Close Reference(reference=w104, error in (no error)=w105) -> ()  [unwired: 1 out]
              n62 = Close Reference(reference=w102, error in (no error)=w101) -> ()  [unwired: 1 out]
              n63 = Close Reference(reference=w96, error in (no error)=w97) -> ()  [unwired: 1 out]
              n64 = case shown="True" w103 {
                tunnel: w89 -> [_ w127]
                tunnel: w91 -> [_ w126]
                tunnel: w88 -> [w121 w125]
                tunnel: w95 -> [_ w124]
                tunnel: [w121 w123] -> w90
                tunnel: w89 -> [_ w122]
                frame False {
                }
                frame True {
                  n65 = case shown="True" w122 {
                    tunnel: w126 -> [_ w129]
                    frame False {
                    }
                    frame True {
                      n66 = Unbundle By Name(w129) -> ("Config Parameters.Re-initilaize"=w132:refnum<vi>)
                      n67 = property class="Bool (strict)"(reference=w132, "Value"=FALSE) -> (reference out=w130:refnum<vi>, error out=w131:errorcluster)  [unwired: 1 in]
                      n68 = Close Reference(reference=w130, error in (no error)=w131) -> ()  [unwired: 1 out]
                    }
                  }
                  n69 = call <vilib>:"Mean PtByPt.vi"("x"=w125, "sample length"=w124, "initialize"=w127) -> ("mean"=w123:dbl)  [unwired: 1 in, 1 out]
                }
              }
              n70 = Unbundle By Name(w91) -> ("Main Screen.Friction Force (N)"=w92:refnum<vi>)
              n71 = property class="DigNum (strict)"(reference=w92, "Value"=w90) -> (reference out=w94:refnum<vi>, error out=w93:errorcluster)  [unwired: 1 in]
              n72 = Close Reference(reference=w94, error in (no error)=w93) -> ()  [unwired: 1 out]
            }
            frame True {
              n73 = Unbundle By Name(w145) -> ("Loading Com Port.FORCE (N)"=w173:refnum<vi>)
              n74 = property class="WFChart (strict)"(reference=w173) -> (reference out=w171:refnum<vi>, error out=w172:errorcluster, "History Data"=w142:dbl[][])  [unwired: 1 in]
              n75 = Unbundle By Name(w145) -> ("Main Screen.Friction Force (N)"=w161:refnum<vi>)
              n76 = Index Array(array=w142, index (col)=1 ("disabled index (col)")) -> (element=w141:dbl[])  [unwired: 1 in]
              n77 = Close Reference(reference=w171, error in (no error)=w172) -> ()  [unwired: 1 out]
              n78 = call-poly <vilib>:"Mean.vi"("X"=w141) -> ("mean"=w170:dbl)  [unwired: 1 out]
              n79 = Unbundle By Name(w145) -> ("Main Screen.CZ FF"=w152:refnum<vi>)
              n80 = Subtract(x=w141, y=w170) -> (x-y=w169:dbl[])
              n81 = property class="DigNum (strict)"(reference=w161) -> (reference out=w163:refnum<vi>, error out=w162:errorcluster, "Value"=w160:dbl)  [unwired: 1 in]
              n82 = property class="Bool (strict)"(reference=w152) -> (reference out=w150:refnum<vi>, error out=w151:errorcluster, "Value"=w149:bool)  [unwired: 1 in]
              n83 = call-poly <vilib>:"RMS.vi"("X"=w169) -> ("rms value"=w167:dbl)  [unwired: 1 out]
              n84 = Unbundle By Name(w145) -> ("Main Screen.zFF"=w159:refnum<vi>)
              n85 = Not A Number/Path/Refnum?(number/path/refnum=w167) -> (NaN/Path/Refnum?=w168:bool)
              n86 = Close Reference(reference=w163, error in (no error)=w162) -> ()  [unwired: 1 out]
              n87 = property class="Bool (strict)"(reference=w159) -> (reference out=w157:refnum<vi>, error out=w158:errorcluster, "Value"=w156:bool)  [unwired: 1 in]
              n88 = Close Reference(reference=w150, error in (no error)=w151) -> ()  [unwired: 1 out]
              n89 = Select(t=w160, s=w168, f=w167) -> (s? t:f=w155:dbl)
              n90 = case shown="True" w149 {
                tunnel: w145 -> [_ w176]
                tunnel: w139 -> [_ w174]
                frame False {
                }
                frame True {
                  n91 = Unbundle By Name(w176) -> ("Main Screen.CZ FF"=w177:refnum<vi>)
                  n92 = property class="Bool (strict)"(reference=w177, "Value"=FALSE) -> (reference out=w179:refnum<vi>, error out=w178:errorcluster)  [unwired: 1 in]
                  n93 = Close Reference(reference=w179, error in (no error)=w178) -> ()  [unwired: 1 out]
                  "Fload 3" <- w174
                }
              }
              n94 = Close Reference(reference=w157, error in (no error)=w158) -> ()  [unwired: 1 out]
              n95 = local read "Fload 2"() -> (w153:dbl)
              n96 = case shown="True" w156 {
                tunnel: w145 -> [_ w182]
                tunnel: w155 -> [_ w180]
                frame False {
                }
                frame True {
                  n97 = Unbundle By Name(w182) -> ("Main Screen.zFF"=w183:refnum<vi>)
                  n98 = property class="Bool (strict)"(reference=w183, "Value"=FALSE) -> (reference out=w185:refnum<vi>, error out=w184:errorcluster)  [unwired: 1 in]
                  n99 = Close Reference(reference=w185, error in (no error)=w184) -> ()  [unwired: 1 out]
                  "Fload 2" <- w180
                }
              }
              n100 = Unbundle By Name(w145) -> ("Main Screen.Friction Force (N)"=w164:refnum<vi>)
              n101 = local read "Fload 3"() -> (w148:dbl)
              n102 = Subtract(x=w155, y=w153) -> (x-y=w154:dbl)
              n103 = Subtract(x=w139, y=w148) -> (x-y=w143:dbl)
              n104 = property class="DigNum (strict)"(reference=w164, "Value"=w154) -> (reference out=w166:refnum<vi>, error out=w165:errorcluster)  [unwired: 1 in]
              n105 = Unbundle By Name(w145) -> ("Main Screen.Cyclic Friction Force (N)"=w146:refnum<vi>)
              n106 = Close Reference(reference=w166, error in (no error)=w165) -> ()  [unwired: 1 out]
              n107 = property class="DigNum (strict)"(reference=w146, "Value"=w143) -> (reference out=w144:refnum<vi>, error out=w147:errorcluster)  [unwired: 1 in]
              n108 = Close Reference(reference=w144, error in (no error)=w147) -> ()  [unwired: 1 out]
            }
          }
          n109 = call-poly <vilib>:"Mean.vi"("X"=w31) -> ("mean"=w80:dbl)  [unwired: 1 out]
          n110 = Negate(x=w80) -> (-x=w67:dbl)
          n111 = Unbundle By Name(w13) -> ("Main Screen.zNL 2"=w71:refnum<vi>)
          n112 = Unbundle By Name(w13) -> ("Motion Module.zNL"=w76:refnum<vi>)
          n113 = property class="Bool (strict)"(reference=w71) -> (reference out=w73:refnum<vi>, error out=w72:errorcluster, "Value"=w69:bool)  [unwired: 1 in]
          n114 = property class="Bool (strict)"(reference=w76) -> (reference out=w74:refnum<vi>, error out=w75:errorcluster, "Value"=w70:bool)  [unwired: 1 in]
          n115 = Close Reference(reference=w73, error in (no error)=w72) -> ()  [unwired: 1 out]
          n116 = Close Reference(reference=w74, error in (no error)=w75) -> ()  [unwired: 1 out]
          n117 = Or(x=w70, y=w69) -> (x .or. y?=w68:bool)
          n118 = case shown="True" w68 {
            tunnel: w67 -> [_ w209]
            tunnel: w13 -> [_ w202]
            frame False {
            }
            frame True {
              w201 = FALSE ("Value")
              n119 = Unbundle By Name(w202) -> ("Main Screen.zNL 2"=w203:refnum<vi>)
              n120 = Unbundle By Name(w202) -> ("Motion Module.zNL"=w208:refnum<vi>)
              n121 = property class="Bool (strict)"(reference=w203, "Value"=w201) -> (reference out=w205:refnum<vi>, error out=w204:errorcluster)  [unwired: 1 in]
              n122 = property class="Bool (strict)"(reference=w208, "Value"=w201) -> (reference out=w206:refnum<vi>, error out=w207:errorcluster)  [unwired: 1 in]
              n123 = Close Reference(reference=w205, error in (no error)=w204) -> ()  [unwired: 1 out]
              n124 = Close Reference(reference=w206, error in (no error)=w207) -> ()  [unwired: 1 out]
              "Zload" <- w209
            }
          }
          n125 = local read "Zload"() -> (w66:dbl)
          n126 = Subtract(x=w67, y=w66) -> (x-y=w61:dbl)
          n127 = Unbundle By Name(w13) -> ("PID.Vertical load (N)"=w79:refnum<vi>)
          n128 = Unbundle By Name(w13) -> ("Config Parameters.Apply Filter (Load)"=w63:refnum<vi>)
          n129 = property class="DigNum (strict)"(reference=w79, "Value"=w61) -> (reference out=w77:refnum<vi>, error out=w78:errorcluster)  [unwired: 1 in]
          n130 = property class="Bool (strict)"(reference=w63) -> (reference out=w65:refnum<vi>, error out=w64:errorcluster, "Value"=w62:bool)  [unwired: 1 in]
          n131 = Close Reference(reference=w77, error in (no error)=w78) -> ()  [unwired: 1 out]
          n132 = Close Reference(reference=w65, error in (no error)=w64) -> ()  [unwired: 1 out]
          n133 = case shown="True" w62 {
            tunnel: w13 -> [_ w197]
            tunnel: w61 -> [w186 w191]
            tunnel: [w186 w188] -> w58
            frame False {
            }
            frame True {
              n134 = Unbundle By Name(w197) -> ("Config Parameters.Filter%"=w200:refnum<vi>)
              n135 = property class="DigNum (strict)"(reference=w200) -> (reference out=w198:refnum<vi>, error out=w199:errorcluster, "Value"=w196:dbl)  [unwired: 1 in]
              n136 = Close Reference(reference=w198, error in (no error)=w199) -> ()  [unwired: 1 out]
              n137 = Multiply(x=w196, y=0.01) -> (x*y=w193:dbl)
              n138 = local read "Load Temp"() -> (w187:dbl)
              n139 = Subtract(x=1.0, y=w193) -> (x-y=w192:dbl)
              n140 = Multiply(x=w191, y=w192) -> (x*y=w190:dbl)
              n141 = Multiply(x=w193, y=w187) -> (x*y=w189:dbl)
              n142 = Add(x=w190, y=w189) -> (x+y=w188:dbl)
            }
          }
          n143 = Not A Number/Path/Refnum?(number/path/refnum=w58) -> (NaN/Path/Refnum?=w60:bool)
          n144 = Unbundle By Name(w13) -> ("Motion Module.NL disp"=w55:refnum<vi>)
          n145 = Unbundle By Name(w13) -> ("Main Screen.NL disp 2"=w54:refnum<vi>)
          n146 = Select(t=0.0, s=w60, f=w58) -> (s? t:f=w51:dbl)
          "Load Temp" <- w51
          n147 = property class="DigNum (strict)"(reference=w55, "Value"=w51) -> (reference out=w57:refnum<vi>, error out=w56:errorcluster)  [unwired: 1 in]
          n148 = property class="DigNum (strict)"(reference=w54, "Value"=w51) -> (reference out=w52:refnum<vi>, error out=w53:errorcluster)  [unwired: 1 in]
          n149 = Close Reference(reference=w57, error in (no error)=w56) -> ()  [unwired: 1 out]
          n150 = Close Reference(reference=w52, error in (no error)=w53) -> ()  [unwired: 1 out]
        }
      }
    }
    frame Error {
    }
  }
  "error out" <- w1
